vi "Picoammeters.vi"(0 "Keithley6487 Current (A)":refnum<vi>, 1 "QUIT":refnum<vi>, 2 "6487 Error":refnum<vi>, 4 "Keithley6487 Voltage (V)":refnum<vi>, 5 "Scan in Progress":refnum<vi>, 6 "6485 Samples/Measurement":refnum<vi>, 7 "Measure 6485":refnum<vi>, 8 "Measure 6487":refnum<vi>, 9 "6485 Error":refnum<vi>, 10 "Keithley6485 Current (A)":refnum<vi>) -> ()   [LabVIEW 2018]
uses:
  <vilib>/Utility/error.llb/DialogType.ctl
panel:
  in  "Picoammeters":T1(tab)
  out "6487 Background Correction":bool caption="Background Correction"
  out "Keithley6485 Current":dbl caption="Current (A)"
  out "Keithley6485 Status":string caption="Status"
  out "Keithley6487 Status":string caption="Status"
  in  "6487 Voltage":dbl caption="Potential (V)" min=-505.0 max=505.0
  out "Keithley6487 Current":dbl caption="Current (A)"
  out "6487 Voltage Feedback":dbl caption="Potential (V)"
  out "6485 Background Correction":bool caption="Background Correction"
  in  "6487 Samples/Measurement Control":u32=1 caption="V" min=1 max=2500 step=1
  out "6487 Samples/Measurement Feedback":u32 caption="Samples/Measurement"
  out "6485 Samples/Measurement Feedback":u32 caption="Samples/Measurement"
  in  "6485 Samples/Measurement Control":u32=1 caption="V" min=1 max=2500 step=1
  out "Keithley6487 Online":bool caption="Online"
  in  "Enable Keithley6487":bool caption="Enable"
  in  "Keithley6485 Port":refnum<visa-resource-name>="COM5"
  out "Keithley6485 Online":bool caption="Online"
  in  "Enable Keithley6485":bool caption="Enable"
  in  "Keithley6487 Port":refnum<visa-resource-name>="COM6"
  in  "6487 ZC Once":bool
  in  "6487 ZC BEM":bool caption="6487"
  in  "6485 CZ Toggle":bool
  in  "6487 CZ Toggle":bool
  in  "6485 ZC Once":bool
  in  "6485 ZC BEM":bool caption="6485"
  in  "Timeout Extension Offset (ms)":u32=1000
  in  "Timeout Extension Rate (ms/sample)":i32=500
  out "Zero Offset 6485":string caption="6485"
  out "Zero Offset 6487":string caption="6487"
  out "6485 Error Message":string=" INSTRUCTIONS:\r\rNormal Use:  When using subVIs that incorporate the error in/error out (or error I/O) structure, place this handler where you want to inform the user of an error, typically at the end of the I/O data path, as the last action of the program.  If the error in error? is ERROR, the handler creates a message describing the error and its source.  If the type of dialog = 1 (default), the message is displayed to the user, who can only acknowedge it.  If the type = 2, the user can acknowledge the message or abort execution; aborting a program with active I/O is not recommended.  If the type = 0, no message is displayed; this is used to process the error programmatically, and the error out cluster elements are wired to individual terminals for that reason.  \r\rOther Use:\n\r\nlocal testing.  To test the error code of a subVI or function that does not have the error I/O structure, you can wire its error code and a source string to the local error code and error source inputs.  If error in error? indicates no error and error code is not equal to 0, the local code and source are substituted for the error in values, and error? is set TRUE (ERROR)."
  out "6487 Error Message":string=" INSTRUCTIONS:\r\rNormal Use:  When using subVIs that incorporate the error in/error out (or error I/O) structure, place this handler where you want to inform the user of an error, typically at the end of the I/O data path, as the last action of the program.  If the error in error? is ERROR, the handler creates a message describing the error and its source.  If the type of dialog = 1 (default), the message is displayed to the user, who can only acknowedge it.  If the type = 2, the user can acknowledge the message or abort execution; aborting a program with active I/O is not recommended.  If the type = 0, no message is displayed; this is used to process the error programmatically, and the error out cluster elements are wired to individual terminals for that reason.  \r\rOther Use:\n\r\nlocal testing.  To test the error code of a subVI or function that does not have the error I/O structure, you can wire its error code and a source string to the local error code and error source inputs.  If error in error? indicates no error and error code is not equal to 0, the local code and source are substituted for the error in values, and error? is set TRUE (ERROR)."
  # "Under normal conditions, 6485 is the Faraday cup and 6487 is the sample."
  # "Measurements continue after window is closed."
  # "We have to set an absolute timeout in ms when reading measurements over a serial line.  This needs to be longer for more samples per measurement.  To avoid setting this to the max possible (which is VERY long), the minimum necessary timeout is calculated for every measurement taken.  A linear model is used, where every sample takes \"Rate\" ms to capture and there is \"Offset\" overhead for each measurement.  The 'correct' values for this model are unkown.  If you are getting timeouts, try increasing either one."
  # "Extra Notes ->"
  # "Serial I/O errors are naturally reported.  The capability to report additional errors returned by the Keithley 6485 picoAmmeter has been added.  Currently, only \"overvoltage\" and \"invalid data\" errors are supported by this VI."
  # "Keithley 6485"
  # "Keithley 6487"
  # "Perform Background\nCheck Once"
  # "Perform Background Check & Correction\nBefore Every Measurement"
  # "Zero Offsets"
  # "Toggle Background Correction"
  # "A background check shunts the input to ground and takes a measurement, thus recording any erroneous zero\noffset.  Enabling background correction subtracts the most recently recorded offset from the data."
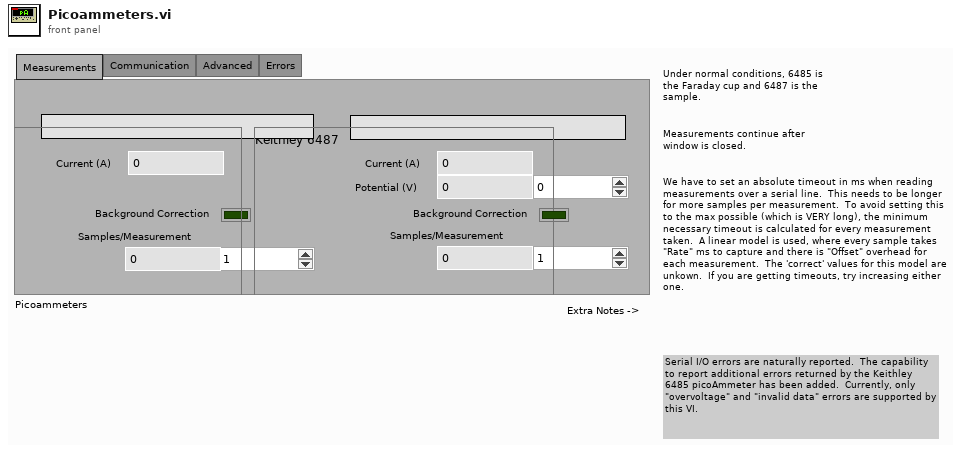
[diagram p1: front panel]
types:
  T1 = enum32{"Measurements", "Communication", "Advanced", "Errors"}
  T2 = typedef "DialogType.ctl" = u16
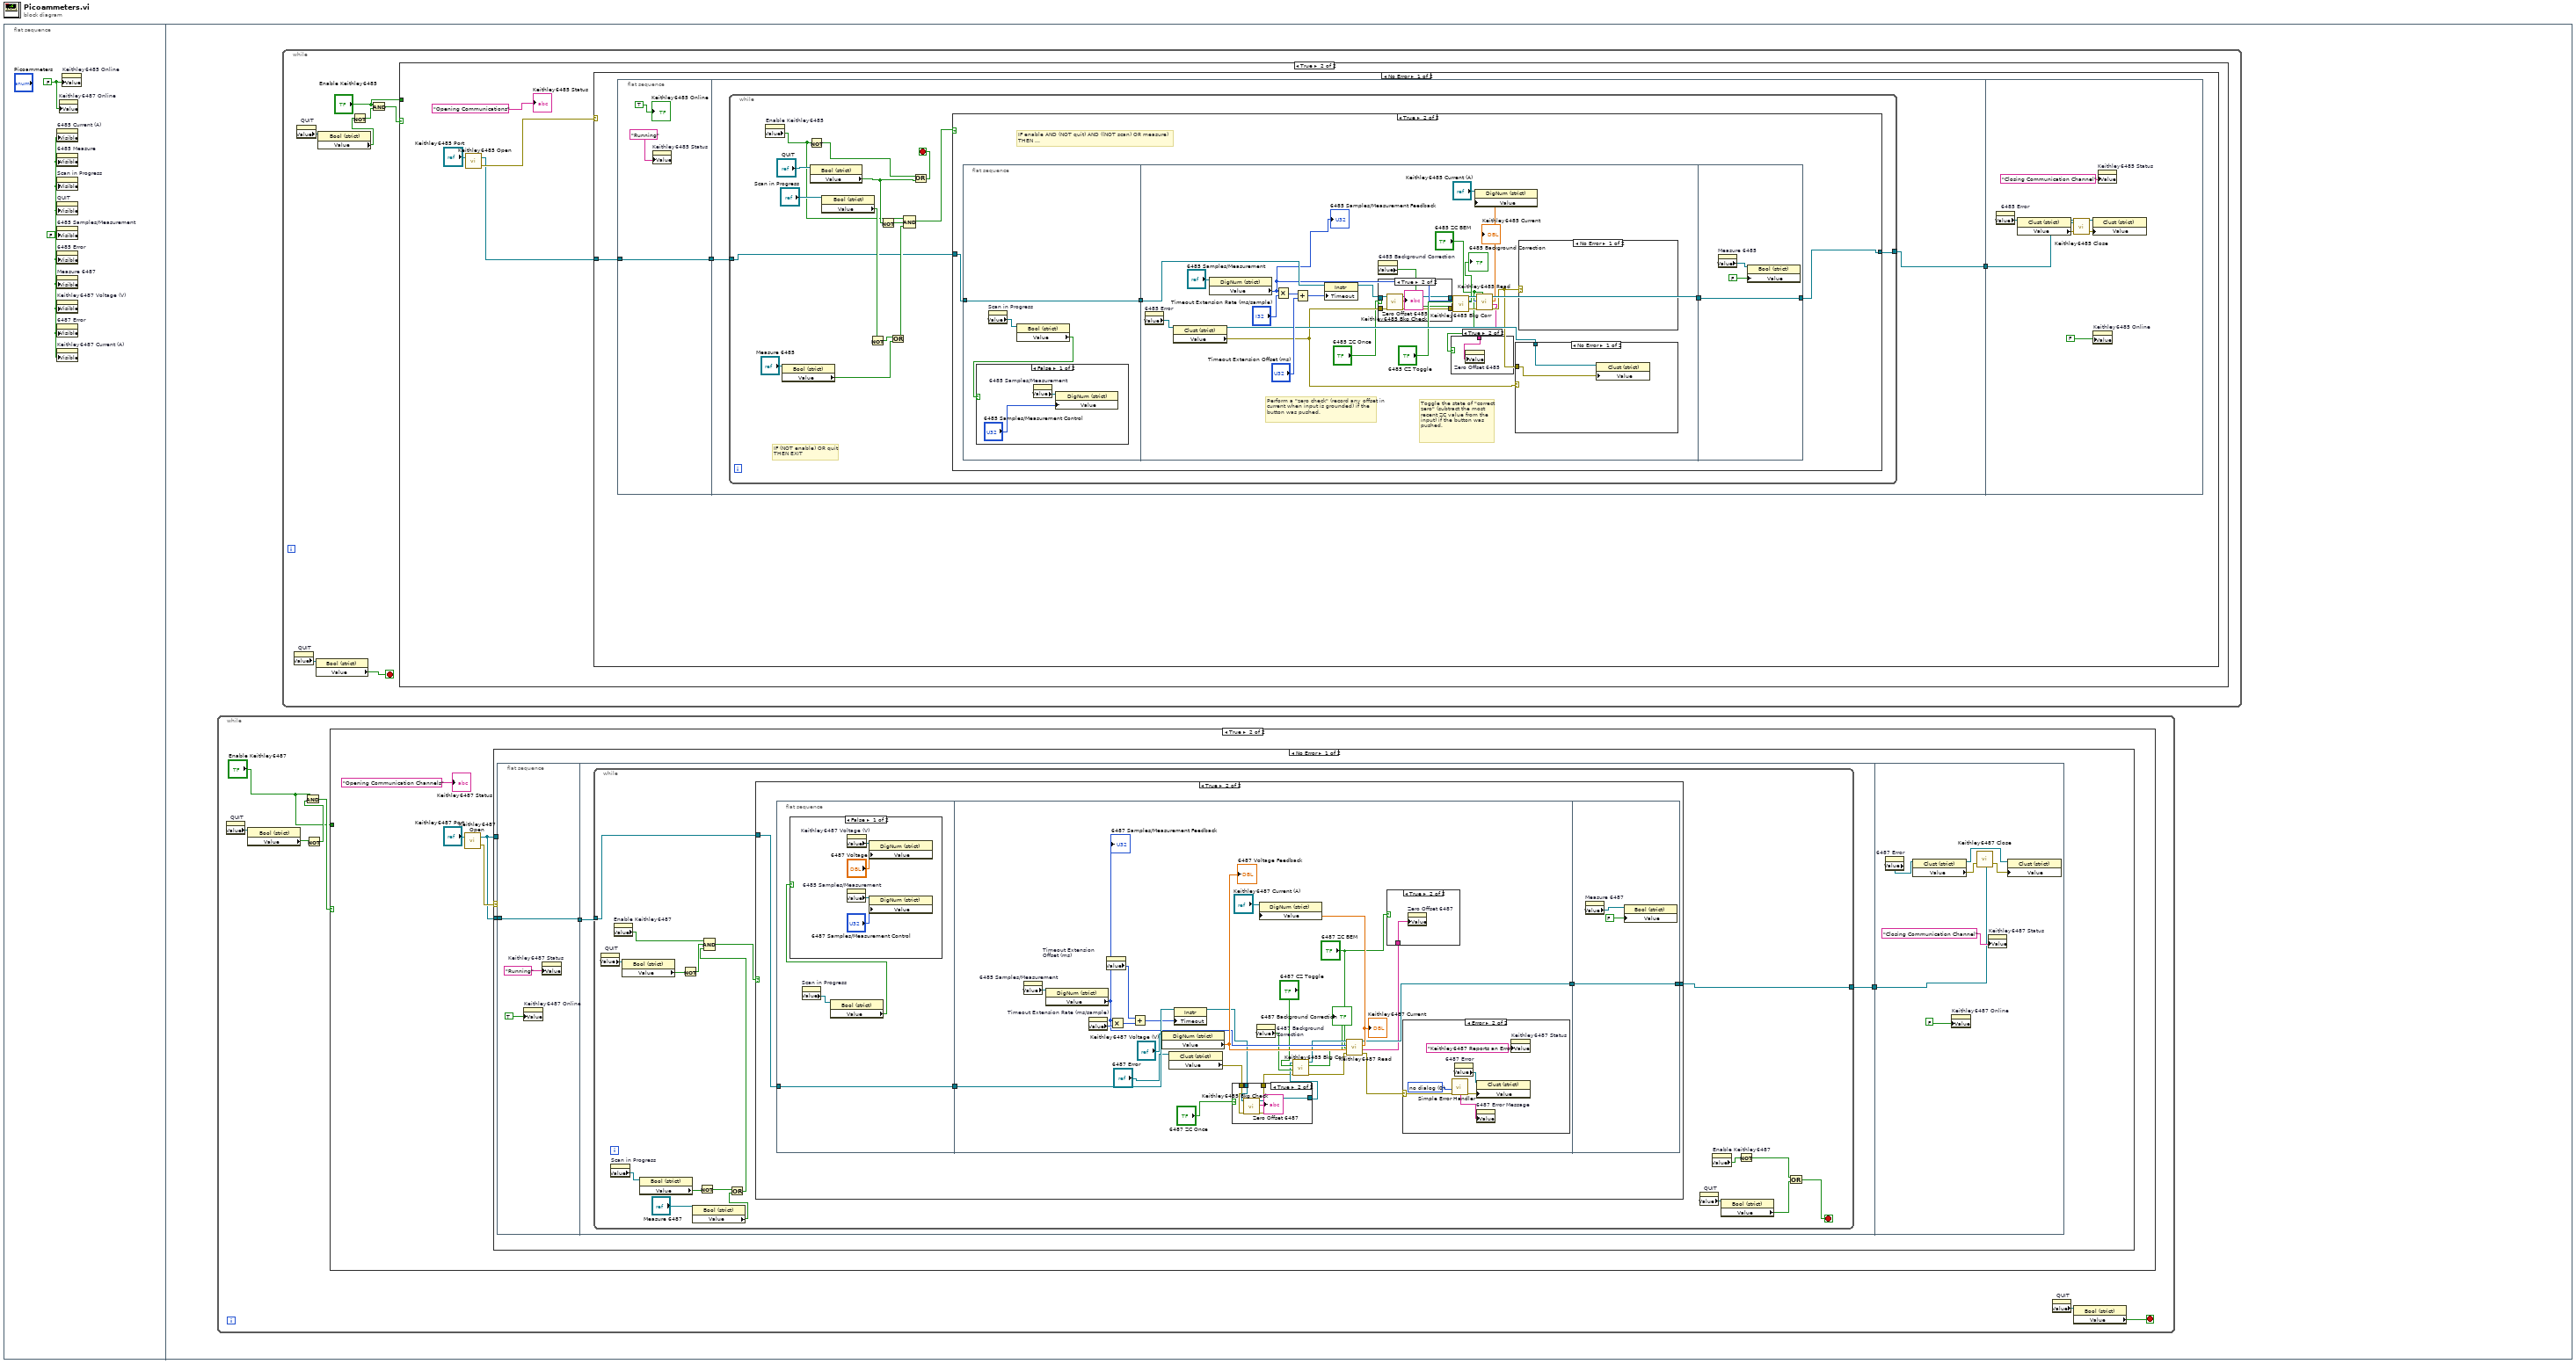
[diagram p0: block diagram]
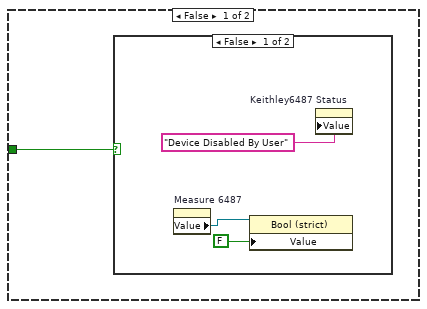
[diagram p2: hidden frame]
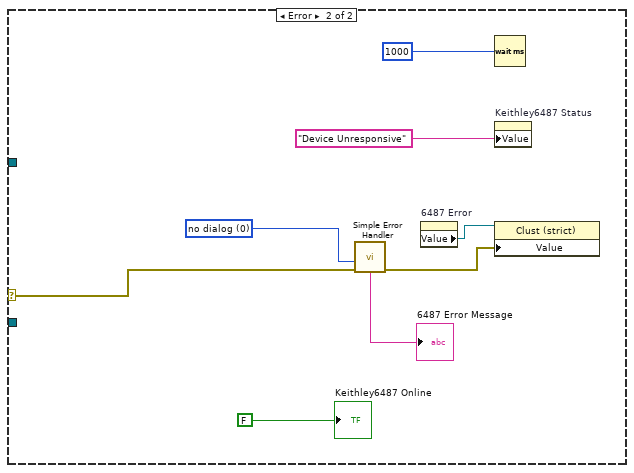
[diagram p9: hidden frame]
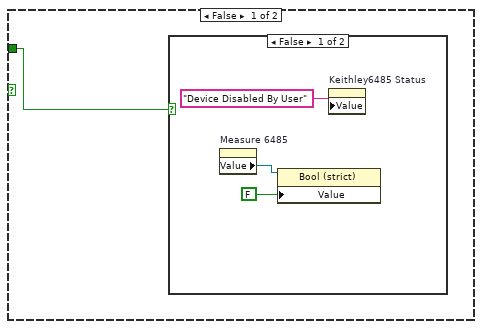
[diagram p10: hidden frame]
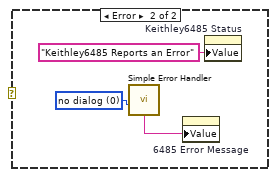
[diagram p17: hidden frame]
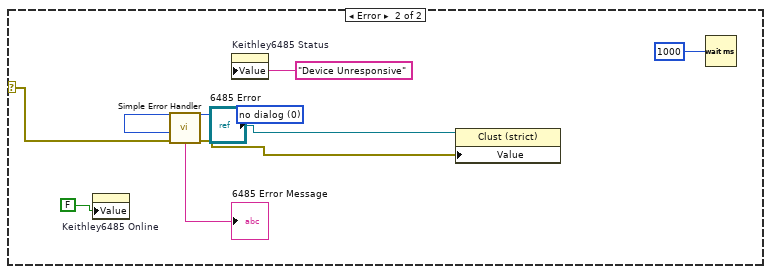
[diagram p18: hidden frame]
diagram:
  n1 = flat-sequence {
    frame #0 {
      w2 = FALSE ("Visible")
      w1 = FALSE ("Online")
      n2 = property on="6485 Current (A)" class="LVObjRef (strict)"("Visible"=w2) -> ()  [unwired: 2 in, 2 out]
      n3 = property on="6485 Measure" class="LVObjRef (strict)"("Visible"=w2) -> ()  [unwired: 2 in, 2 out]
      n4 = property on="Scan in Progress" class="LVObjRef (strict)"("Visible"=w2) -> ()  [unwired: 2 in, 2 out]
      n5 = property on="QUIT" class="LVObjRef (strict)"("Visible"=w2) -> ()  [unwired: 2 in, 2 out]
      n6 = property on="6485 Samples/Measurement" class="LVObjRef (strict)"("Visible"=w2) -> ()  [unwired: 2 in, 2 out]
      n7 = property on="6485 Error" class="LVObjRef (strict)"("Visible"=w2) -> ()  [unwired: 2 in, 2 out]
      n8 = property on="Measure 6487" class="LVObjRef (strict)"("Visible"=w2) -> ()  [unwired: 2 in, 2 out]
      n9 = property on="Keithley6487 Voltage (V)" class="LVObjRef (strict)"("Visible"=w2) -> ()  [unwired: 2 in, 2 out]
      n10 = property on="6487 Error" class="LVObjRef (strict)"("Visible"=w2) -> ()  [unwired: 2 in, 2 out]
      n11 = property on="Keithley6487 Current (A)" class="LVObjRef (strict)"("Visible"=w2) -> ()  [unwired: 2 in, 2 out]
      n12 = property on="Keithley6487 Online" class="Bool (strict)"("Value"=w1) -> ()  [unwired: 2 in, 2 out]
      n13 = property on="Keithley6485 Online" class="Bool (strict)"("Value"=w1) -> ()  [unwired: 2 in, 2 out]
    }
    frame #1 {
      n14 = while {
        stop <- w4 stop-if-true
        n15 = property on="QUIT" class="LVObjRef (strict)"() -> ("Value"=w9:refnum<vi>)  [unwired: 2 in, 2 out]
        n16 = property on="Property Node" class="Bool (strict)"(reference=w9) -> ("Value"=w8:bool)  [unwired: 1 in, 2 out]
        n17 = Not(x=w8) -> (.not. x?=w7:bool)
        n18 = And(x="Enable Keithley6487", y=w7) -> (x .and. y?=w6:bool)
        n19 = case shown="True" w6 {
          tunnel: "Enable Keithley6487" -> [w10 _]
          frame False {
            n20 = case shown="False" w10 {
              frame False {
                n21 = property on="Measure 6487" class="LVObjRef (strict)"() -> ("Value"=w13:refnum<vi>)  [unwired: 2 in, 2 out]
                n22 = property on="Property Node" class="Bool (strict)"(reference=w13, "Value"=FALSE) -> ()  [unwired: 1 in, 2 out]
                n23 = property on="Keithley6487 Status" class="Str"("Value"="Device Disabled By User" ("Keithley6487 Status")) -> ()  [unwired: 2 in, 2 out]
              }
              frame True {
              }
            }
          }
          frame True {
            n24 = call "Keithley6487 Open.vi"("VISA resource name"="Keithley6487 Port") -> ("Error out"=w16:errorcluster, "VISA out"=w14:refnum<visa-resource-name>)  [unwired: 1 in]
            n25 = case shown="No Error" w16 {
              selector: w16 -> [_ w110]
              tunnel: w14 -> [_ _]
              tunnel: w14 -> [w20 _]
              frame No Error {
                n26 = flat-sequence {
                  tunnel: w20 -> [w21]
                  tunnel: [w21] -> w19
                  tunnel: w19 -> [w24]
                  tunnel: [w25] -> w18
                  tunnel: w18 -> [w100]
                  frame #0 {
                    n27 = property on="Keithley6487 Online" class="Bool (strict)"("Value"=TRUE ("Keithley6487 Online")) -> ()  [unwired: 2 in, 2 out]
                    n28 = property on="Keithley6487 Status" class="Str"("Value"="Running" ("Keithley6487 Status")) -> ()  [unwired: 2 in, 2 out]
                  }
                  frame #1 {
                    n29 = while {
                      tunnel: w24 -> [w28]
                      tunnel: [w26] -> w25
                      stop <- w39 stop-if-true
                      n30 = property on="QUIT" class="LVObjRef (strict)"() -> ("Value"=w37:refnum<vi>)  [unwired: 2 in, 2 out]
                      n31 = property on="Scan in Progress" class="LVObjRef (strict)"() -> ("Value"=w34:refnum<vi>)  [unwired: 2 in, 2 out]
                      n32 = property on="Enable Keithley6487" class="Bool (strict)"() -> ("Value"=w38:bool)  [unwired: 2 in, 2 out]
                      n33 = property on="Property Node" class="Bool (strict)"(reference=w37) -> ("Value"=w36:bool)  [unwired: 1 in, 2 out]
                      n34 = property on="Property Node" class="Bool (strict)"(reference=w34) -> ("Value"=w33:bool)  [unwired: 1 in, 2 out]
                      n35 = Not(x=w36) -> (.not. x?=w35:bool)
                      n36 = property on="Property Node" class="Bool (strict)"(reference="Measure 6487") -> ("Value"=w31:bool)  [unwired: 1 in, 2 out]
                      n37 = Not(x=w33) -> (.not. x?=w32:bool)
                      n38 = Or(x=w32, y=w31) -> (x .or. y?=w30:bool)
                      n39 = Compound Arithmetic op=AND(w38, w35, w30) -> (w29:bool)
                      n40 = case shown="True" w29 {
                        tunnel: w28 -> [w44 w48]
                        tunnel: [w44 w46] -> w26
                        frame False {
                        }
                        frame True {
                          n41 = flat-sequence {
                            tunnel: w48 -> [w51]
                            tunnel: [w51] -> w47
                            tunnel: w47 -> [w81]
                            tunnel: [w69] -> w45
                            tunnel: [w98] -> w46
                            tunnel: w45 -> [w98]
                            frame #0 {
                              n42 = property on="Scan in Progress" class="LVObjRef (strict)"() -> ("Value"=w50:refnum<vi>)  [unwired: 2 in, 2 out]
                              n43 = property on="Property Node" class="Bool (strict)"(reference=w50) -> ("Value"=w49:bool)  [unwired: 1 in, 2 out]
                              n44 = case shown="False" w49 {
                                frame False {
                                n45 = property on="6485 Samples/Measurement" class="LVObjRef (strict)"() -> ("Value"=w53:refnum<vi>)  [unwired: 2 in, 2 out]
                                n46 = property on="Keithley6487 Voltage (V)" class="LVObjRef (strict)"() -> ("Value"=w55:refnum<vi>)  [unwired: 2 in, 2 out]
                                n47 = property on="Property Node" class="DigNum (strict)"(reference=w55, "Value"="6487 Voltage") -> ()  [unwired: 1 in, 2 out]
                                n48 = property on="Property Node" class="DigNum (strict)"(reference=w53, "Value"="6487 Samples/Measurement Control") -> ()  [unwired: 1 in, 2 out]
                                }
                                frame True {
                                }
                              }
                            }
                            frame #1 {
                              n49 = property on="6485 Samples/Measurement" class="LVObjRef (strict)"() -> ("Value"=w80:refnum<vi>)  [unwired: 2 in, 2 out]
                              n50 = property on="Property Node" class="DigNum (strict)"(reference=w80) -> ("Value"=w71:i32)  [unwired: 1 in, 2 out]
                              "6487 Samples/Measurement Feedback" <- w71
                              n51 = property on="Timeout Extension Rate (ms/sample)" class="DigNum (strict)"() -> ("Value"=w79:i32)  [unwired: 2 in, 2 out]
                              n52 = property on="Timeout Extension Offset (ms)" class="DigNum (strict)"() -> ("Value"=w77:u32)  [unwired: 2 in, 2 out]
                              n53 = Multiply(x=w71, y=w79) -> (x*y=w78:i32)
                              n54 = Add(x=w77, y=w78) -> (x+y=w76:u32)
                              n55 = property on="Property Node" class="DigNum (strict)"(reference="Keithley6487 Voltage (V)") -> ("Value"=w72:dbl)  [unwired: 1 in, 2 out]
                              "6487 Voltage Feedback" <- w72
                              n56 = property on="Property Node" class="Clust (strict)"(reference="6487 Error") -> ("Value"=w66:errorcluster)  [unwired: 1 in, 2 out]
                              n57 = property class="Instr"(reference=w81, "Timeout"=w76) -> (reference out=w65:refnum<visa-resource-name>)  [unwired: 1 in, 1 out]
                              n58 = case shown="True" "6487 ZC Once" {
                                tunnel: w66 -> [w83 w88]
                                tunnel: [w83 w86] -> w58
                                tunnel: w65 -> [w84 w89]
                                tunnel: [w84 w87] -> w59
                                frame False {
                                }
                                frame True {
                                n59 = call "Keithley6485 Bkg Check.vi"("error in"=w88, "VISA in"=w89) -> ("error out"=w86:errorcluster, "Zero Offset"=→"Zero Offset 6487":string, "VISA out"=w87:refnum<visa-resource-name>)  [unwired: 7 in]
                                }
                              }
                              n60 = property on="6487 Background Correction" class="Bool (strict)"() -> ("Value"=w60:bool)  [unwired: 2 in, 2 out]
                              n61 = call "Keithley6485 Bkg Corr.vi"("error in"=w58, "ZC Before"=w60, "ZC Toggle"="6487 CZ Toggle", "VISA in"=w59) -> ("error out"=w64:errorcluster, "ZC After"=→"6487 Background Correction":bool, "VISA out"=w63:refnum<visa-resource-name>)  [unwired: 5 in]
                              n62 = call "Keithley6487 Read.vi"("Enable Zero Correction"="6487 ZC BEM", "error in"=w64, "Voltage (V)"=w72, "Sample per measurement"=w71, "VISA in"=w63) -> ("error out"=w70:errorcluster, "Zero Offset"=w56:string, "Current (A)"=w73:dbl, "VISA out"=w69:refnum<visa-resource-name>)  [unwired: 3 in]
                              "Keithley6487 Current" <- w73
                              n63 = property on="Property Node" class="DigNum (strict)"(reference="Keithley6487 Current (A)", "Value"=w73) -> ()  [unwired: 1 in, 2 out]
                              n64 = case shown="True" "6487 ZC BEM" {
                                tunnel: w56 -> [_ w82]
                                frame False {
                                }
                                frame True {
                                n65 = property on="Zero Offset 6487" class="Str"("Value"=w82) -> ()  [unwired: 2 in, 2 out]
                                }
                              }
                              n66 = case shown="Error" w70 {
                                selector: w70 -> [_ w95]
                                frame No Error {
                                }
                                frame Error {
                                w94 = T2 0 items=["no dialog", "OK message", "continue or stop message", "OK message + warnings", "continue/stop + warnings"] ("type of dialog (OK msg:1)")
                                n67 = call <vilib>:"Simple Error Handler.vi"("type of dialog (OK msg:1)"=w94, "error in (no error)"=w95) -> ("error out"=w92:errorcluster, "message"=w93:string)  [unwired: 3 in, 3 out]
                                n68 = property on="6487 Error" class="LVObjRef (strict)"() -> ("Value"=w91:refnum<vi>)  [unwired: 2 in, 2 out]
                                n69 = property on="Property Node" class="Clust (strict)"(reference=w91, "Value"=w92) -> ()  [unwired: 1 in, 2 out]
                                n70 = property on="6487 Error Message" class="Str"("Value"=w93) -> ()  [unwired: 2 in, 2 out]
                                n71 = property on="Keithley6487 Status" class="Str"("Value"="Keithley6487 Reports an Error" ("Keithley6487 Status")) -> ()  [unwired: 2 in, 2 out]
                                }
                              }
                            }
                            frame #2 {
                              n72 = property on="Measure 6487" class="LVObjRef (strict)"() -> ("Value"=w97:refnum<vi>)  [unwired: 2 in, 2 out]
                              n73 = property on="Property Node" class="Bool (strict)"(reference=w97, "Value"=FALSE) -> ()  [unwired: 1 in, 2 out]
                            }
                          }
                        }
                      }
                      n74 = property on="QUIT" class="LVObjRef (strict)"() -> ("Value"=w42:refnum<vi>)  [unwired: 2 in, 2 out]
                      n75 = property on="Enable Keithley6487" class="Bool (strict)"() -> ("Value"=w43:bool)  [unwired: 2 in, 2 out]
                      n76 = property on="Property Node" class="Bool (strict)"(reference=w42) -> ("Value"=w40:bool)  [unwired: 1 in, 2 out]
                      n77 = Not(x=w43) -> (.not. x?=w41:bool)
                      n78 = Or(x=w41, y=w40) -> (x .or. y?=w39:bool)
                    }
                  }
                  frame #2 {
                    n79 = property on="6487 Error" class="LVObjRef (strict)"() -> ("Value"=w105:refnum<vi>)  [unwired: 2 in, 2 out]
                    n80 = property on="Property Node" class="Clust (strict)"(reference=w105) -> (reference out=w103:refnum<vi>, "Value"=w104:errorcluster)  [unwired: 1 in, 1 out]
                    n81 = property on="Keithley6487 Online" class="Bool (strict)"("Value"=FALSE) -> ()  [unwired: 2 in, 2 out]
                    n82 = call "Keithley6487 Close.vi"("error in"=w104, "VISA in"=w100) -> ("error out"=w102:errorcluster)  [unwired: 1 in]
                    n83 = property on="Keithley6487 Status" class="Str"("Value"="Closing Communication Channel") -> ()  [unwired: 2 in, 2 out]
                    n84 = property on="Property Node" class="Clust (strict)"(reference=w103, "Value"=w102) -> ()  [unwired: 1 in, 2 out]
                  }
                }
              }
              frame Error {
                w111 = T2 0 items=["no dialog", "OK message", "continue or stop message", "OK message + warnings", "continue/stop + warnings"] ("type of dialog (OK msg:1)")
                n85 = call <vilib>:"Simple Error Handler.vi"("type of dialog (OK msg:1)"=w111, "error in (no error)"=w110) -> ("error out"=w106:errorcluster, "message"=→"6487 Error Message":string)  [unwired: 3 in, 3 out]
                n86 = property on="6487 Error" class="LVObjRef (strict)"() -> ("Value"=w107:refnum<vi>)  [unwired: 2 in, 2 out]
                n87 = Wait (ms)(milliseconds to wait=u32 1000) -> ()  [unwired: 1 out]
                n88 = property on="Keithley6487 Status" class="Str"("Value"="Device Unresponsive" ("Keithley6487 Status")) -> ()  [unwired: 2 in, 2 out]
                n89 = property on="Property Node" class="Clust (strict)"(reference=w107, "Value"=w106) -> ()  [unwired: 1 in, 2 out]
                "Keithley6487 Online" <- FALSE ("Keithley6487 Online")
              }
            }
            "Keithley6487 Status" <- "Opening Communication Channels" ("Keithley6487 Status")
          }
        }
        n90 = property on="QUIT" class="LVObjRef (strict)"() -> ("Value"=w5:refnum<vi>)  [unwired: 2 in, 2 out]
        n91 = property on="Property Node" class="Bool (strict)"(reference=w5) -> ("Value"=w4:bool)  [unwired: 1 in, 2 out]
      }
      n92 = while {
        stop <- w115 stop-if-true
        n93 = property on="QUIT" class="LVObjRef (strict)"() -> ("Value"=w116:refnum<vi>)  [unwired: 2 in, 2 out]
        n94 = property on="QUIT" class="LVObjRef (strict)"() -> ("Value"=w119:refnum<vi>)  [unwired: 2 in, 2 out]
        n95 = property on="Property Node" class="Bool (strict)"(reference=w116) -> ("Value"=w115:bool)  [unwired: 1 in, 2 out]
        n96 = property on="Property Node" class="Bool (strict)"(reference=w119) -> ("Value"=w117:bool)  [unwired: 1 in, 2 out]
        n97 = Not(x=w117) -> (.not. x?=w118:bool)
        n98 = And(x="Enable Keithley6485", y=w118) -> (x .and. y?=w120:bool)
        n99 = case shown="True" w120 {
          tunnel: "Enable Keithley6485" -> [w121 _]
          frame False {
            n100 = case shown="False" w121 {
              frame False {
                n101 = property on="Measure 6485" class="LVObjRef (strict)"() -> ("Value"=w123:refnum<vi>)  [unwired: 2 in, 2 out]
                n102 = property on="Property Node" class="Bool (strict)"(reference=w123, "Value"=FALSE) -> ()  [unwired: 1 in, 2 out]
                n103 = property on="Keithley6485 Status" class="Str"("Value"="Device Disabled By User" ("Keithley6485 Status")) -> ()  [unwired: 2 in, 2 out]
              }
              frame True {
              }
            }
          }
          frame True {
            n104 = call "Keithley6485 Open.vi"("VISA resource name"="Keithley6485 Port") -> ("Error out"=w127:errorcluster, "VISA out"=w125:refnum<visa-resource-name>)  [unwired: 1 in]
            n105 = case shown="No Error" w127 {
              selector: w127 -> [_ w216]
              tunnel: w125 -> [w131 _]
              frame No Error {
                n106 = flat-sequence {
                  tunnel: w131 -> [w132]
                  tunnel: [w132] -> w130
                  tunnel: w130 -> [w136]
                  tunnel: [w135] -> w129
                  tunnel: w129 -> [w204]
                  frame #0 {
                    n107 = property on="Keithley6485 Status" class="Str"("Value"="Running") -> ()  [unwired: 2 in, 2 out]
                    "Keithley6485 Online" <- TRUE ("Online")
                  }
                  frame #1 {
                    n108 = while {
                      tunnel: [w151] -> w135
                      tunnel: w136 -> [w137]
                      stop <- w148 stop-if-true
                      # "IF (NOT enable) OR quit\nTHEN EXIT"
                      n109 = property on="Enable Keithley6485" class="Bool (strict)"() -> ("Value"=w138:bool)  [unwired: 2 in, 2 out]
                      n110 = property on="Property Node" class="Bool (strict)"(reference="Measure 6485") -> ("Value"=w141:bool)  [unwired: 1 in, 2 out]
                      n111 = Not(x=w138) -> (.not. x?=w147:bool)
                      n112 = property on="Property Node" class="Bool (strict)"(reference="QUIT") -> ("Value"=w145:bool)  [unwired: 1 in, 2 out]
                      n113 = property on="Property Node" class="Bool (strict)"(reference="Scan in Progress") -> ("Value"=w144:bool)  [unwired: 1 in, 2 out]
                      n114 = Not(x=w144) -> (.not. x?=w143:bool)
                      n115 = Not(x=w145) -> (.not. x?=w146:bool)
                      n116 = Or(x=w143, y=w141) -> (x .or. y?=w140:bool)
                      n117 = Compound Arithmetic op=AND(w138, w146, w140) -> (w139:bool)
                      n118 = Or(x=w147, y=w145) -> (x .or. y?=w148:bool)
                      n119 = case shown="True" w139 {
                        tunnel: [w152 w154] -> w151
                        tunnel: w137 -> [w152 w153]
                        frame False {
                        }
                        frame True {
                          # "IF enable AND (NOT quit) AND ((NOT scan) OR measure) \nTHEN ..."
                          n120 = flat-sequence {
                            tunnel: w153 -> [w159]
                            tunnel: [w159] -> w156
                            tunnel: w156 -> [w177]
                            tunnel: [w186] -> w155
                            tunnel: [w202] -> w154
                            tunnel: w155 -> [w202]
                            frame #0 {
                              n121 = property on="Scan in Progress" class="LVObjRef (strict)"() -> ("Value"=w158:refnum<vi>)  [unwired: 2 in, 2 out]
                              n122 = property on="Property Node" class="Bool (strict)"(reference=w158) -> ("Value"=w157:bool)  [unwired: 1 in, 2 out]
                              n123 = case shown="False" w157 {
                                frame False {
                                n124 = property on="6485 Samples/Measurement" class="LVObjRef (strict)"() -> ("Value"=w161:refnum<vi>)  [unwired: 2 in, 2 out]
                                n125 = property on="Property Node" class="DigNum (strict)"(reference=w161, "Value"="6485 Samples/Measurement Control") -> ()  [unwired: 1 in, 2 out]
                                }
                                frame True {
                                }
                              }
                            }
                            frame #1 {
                              # "Toggle the state of \"correct zero\" (subtract the most recent ZC value from the input) if the button was pushed."
                              # "Perform a \"zero check\" (record any offset in current when input is grounded) if the button was pushed."
                              n126 = property on="6485 Error" class="LVObjRef (strict)"() -> ("Value"=w178:refnum<vi>)  [unwired: 2 in, 2 out]
                              n127 = property on="Property Node" class="Clust (strict)"(reference=w178) -> (reference out=w176:refnum<vi>, "Value"=w173:errorcluster)  [unwired: 1 in, 1 out]
                              n128 = property on="Property Node" class="DigNum (strict)"(reference="6485 Samples/Measurement") -> ("Value"=w164:i32)  [unwired: 1 in, 2 out]
                              "6485 Samples/Measurement Feedback" <- w164
                              n129 = Multiply(x=w164, y="Timeout Extension Rate (ms/sample)") -> (x*y=w185:i32)
                              n130 = Add(x=w185, y="Timeout Extension Offset (ms)") -> (x+y=w183:u32)
                              n131 = property class="Instr"(reference=w177, "Timeout"=w183) -> (reference out=w174:refnum<visa-resource-name>)  [unwired: 1 in, 1 out]
                              n132 = property on="6485 Background Correction" class="Bool (strict)"() -> ("Value"=w165:bool)  [unwired: 2 in, 2 out]
                              n133 = case shown="True" "6485 ZC Once" {
                                tunnel: [w189 w194] -> w170
                                tunnel: w174 -> [w189 w193]
                                tunnel: [w188 w192] -> w168
                                tunnel: w173 -> [w188 w191]
                                frame False {
                                }
                                frame True {
                                n134 = call "Keithley6485 Bkg Check.vi"("error in"=w191, "VISA in"=w193) -> ("error out"=w192:errorcluster, "Zero Offset"=→"Zero Offset 6485":string, "VISA out"=w194:refnum<visa-resource-name>)  [unwired: 7 in]
                                }
                              }
                              n135 = call "Keithley6485 Bkg Corr.vi"("error in"=w168, "ZC Before"=w165, "ZC Toggle"="6485 CZ Toggle", "VISA in"=w170) -> ("error out"=w169:errorcluster, "ZC After"=→"6485 Background Correction":bool, "VISA out"=w171:refnum<visa-resource-name>)  [unwired: 5 in]
                              n136 = call "Keithley6485 Read.vi"("Enable Zero Correction"="6485 ZC BEM", "error in"=w169, "Sample per measurement"=w164, "VISA in"=w171) -> ("error out"=w175:errorcluster, "Zero Offset"=w162:string, "Current (A)"=w181:dbl, "VISA out"=w186:refnum<visa-resource-name>)  [unwired: 4 in]
                              "Keithley6485 Current" <- w181
                              n137 = case shown="True" "6485 ZC BEM" {
                                tunnel: w162 -> [_ w187]
                                frame False {
                                }
                                frame True {
                                n138 = property on="Zero Offset 6485" class="Str"("Value"=w187) -> ()  [unwired: 2 in, 2 out]
                                }
                              }
                              n139 = property on="Property Node" class="DigNum (strict)"(reference="Keithley6485 Current (A)", "Value"=w181) -> ()  [unwired: 1 in, 2 out]
                              n140 = case shown="No Error" w173 {
                                tunnel: w176 -> [w196 _]
                                tunnel: w175 -> [w195 _]
                                frame No Error {
                                n141 = property on="Property Node" class="Clust (strict)"(reference=w196, "Value"=w195) -> ()  [unwired: 1 in, 2 out]
                                }
                                frame Error {
                                }
                              }
                              n142 = case shown="No Error" w175 {
                                frame No Error {
                                }
                                frame Error {
                                w198 = T2 0 items=["no dialog", "OK message", "continue or stop message", "OK message + warnings", "continue/stop + warnings"] ("type of dialog (OK msg:1)")
                                n143 = call <vilib>:"Simple Error Handler.vi"("type of dialog (OK msg:1)"=w198) -> ("message"=w197:string)  [unwired: 4 in, 4 out]
                                n144 = property on="6485 Error Message" class="Str"("Value"=w197) -> ()  [unwired: 2 in, 2 out]
                                n145 = property on="Keithley6485 Status" class="Str"("Value"="Keithley6485 Reports an Error" ("Status")) -> ()  [unwired: 2 in, 2 out]
                                }
                              }
                            }
                            frame #2 {
                              n146 = property on="Measure 6485" class="LVObjRef (strict)"() -> ("Value"=w201:refnum<vi>)  [unwired: 2 in, 2 out]
                              n147 = property on="Property Node" class="Bool (strict)"(reference=w201, "Value"=FALSE) -> ()  [unwired: 1 in, 2 out]
                            }
                          }
                        }
                      }
                    }
                  }
                  frame #2 {
                    n148 = property on="6485 Error" class="LVObjRef (strict)"() -> ("Value"=w208:refnum<vi>)  [unwired: 2 in, 2 out]
                    n149 = property on="Property Node" class="Clust (strict)"(reference=w208) -> (reference out=w209:refnum<vi>, "Value"=w207:errorcluster)  [unwired: 1 in, 1 out]
                    n150 = call "Keithley6485 Close.vi"("error in"=w207, "VISA in"=w204) -> ("error out"=w206:errorcluster)  [unwired: 1 in]
                    n151 = property on="Property Node" class="Clust (strict)"(reference=w209, "Value"=w206) -> ()  [unwired: 1 in, 2 out]
                    n152 = property on="Keithley6485 Online" class="Bool (strict)"("Value"=FALSE) -> ()  [unwired: 2 in, 2 out]
                    n153 = property on="Keithley6485 Status" class="Str"("Value"="Closing Communication Channel") -> ()  [unwired: 2 in, 2 out]
                  }
                }
              }
              frame Error {
                w215 = T2 0 items=["no dialog", "OK message", "continue or stop message", "OK message + warnings", "continue/stop + warnings"] ("type of dialog (OK msg:1)")
                n154 = property on="Keithley6485 Online" class="Bool (strict)"("Value"=FALSE ("Online")) -> ()  [unwired: 2 in, 2 out]
                n155 = call <vilib>:"Simple Error Handler.vi"("type of dialog (OK msg:1)"=w215, "error in (no error)"=w216) -> ("error out"=w213:errorcluster, "message"=→"6485 Error Message":string)  [unwired: 3 in, 3 out]
                n156 = property on="Keithley6485 Status" class="Str"("Value"="Device Unresponsive") -> ()  [unwired: 2 in, 2 out]
                n157 = property on="Property Node" class="Clust (strict)"(reference="6485 Error", "Value"=w213) -> ()  [unwired: 1 in, 2 out]
                n158 = Wait (ms)(milliseconds to wait=u32 1000) -> ()  [unwired: 1 out]
              }
            }
            "Keithley6485 Status" <- "Opening Communications" ("Value")
          }
        }
      }
    }
  }
